vi "Write Delay.vi"(8 "error in (no error)":errorcluster, 10 "Delay":dbl, 11 "Cheat in":refnum<class "Cheat.lvclass">) -> (0 "error out":errorcluster, 3 "Cheat out":refnum<class "Cheat.lvclass">)   [LabVIEW 2019, in "RT_Game.lvlib" / "Cheat.lvclass"]
uses:
  Cheat.lvclass
  Cheat.lvclass/Cheat.ctl
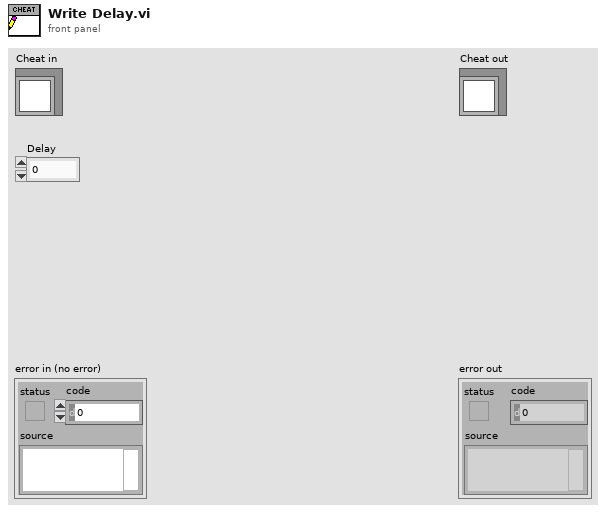
[diagram p1: front panel]
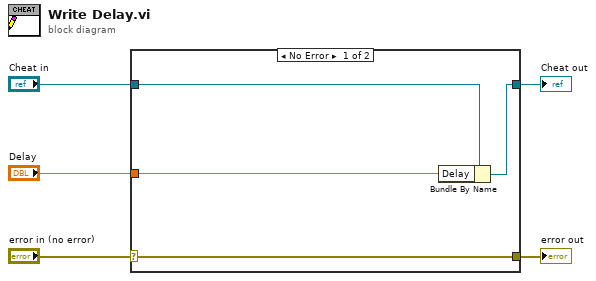
[diagram p0: block diagram]
diagram:
  n1 = case shown="No Error" "error in (no error)" {
    selector: "error in (no error)" -> [w9 w10]
    tunnel: [w9 w10] -> w4
    tunnel: [w7 w11] -> w2
    tunnel: "Cheat in" -> [w8 w11]
    tunnel: "Delay" -> [w6 _]
    frame No Error {
      n2 = Bundle By Name(cluster=w8, "Delay"=w6) -> (w7:refnum<class "Cheat.lvclass">)
    }
    frame Error {
    }
  }
  "error out" <- w4
  "Cheat out" <- w2
